vi "fpga_ResamlingCore.vi"(0 "data in":i32, 1 "Channel number":u8, 2 "timestamp":fxp<+,64,32> format="%.42g", 5 "input data valid":bool, 7 "reference in":fxp<+/-,24,3>, 9 "input reference valid":bool, 11 "interpolation factor":u16=192, 12 "Ready for output":bool, 13 "Fnom":T1 items=["Fnom=50Hz", "Fnom=60Hz"]) -> (4 "Resample data and time":T2, 8 "resampling valid":bool, 10 "output valid":bool, 14 "Ready for reference input":bool, 15 "FIFO timeout?":bool)   [LabVIEW 2011, in "NI_EP_Resample_FPGA.lvlib"]
uses:
  <vilib>/addons/Electrical Power/PQ/Resampling/NI_EP_Resample_FPGA.lvlib
  <vilib>/addons/Electrical Power/PQ/Resampling/FPGA/subVIs/fpga_Resampled.ctl
  <vilib>/addons/Electrical Power/PQ/Resampling/FPGA/subVIs/fpga_Typedef Fnom.ctl
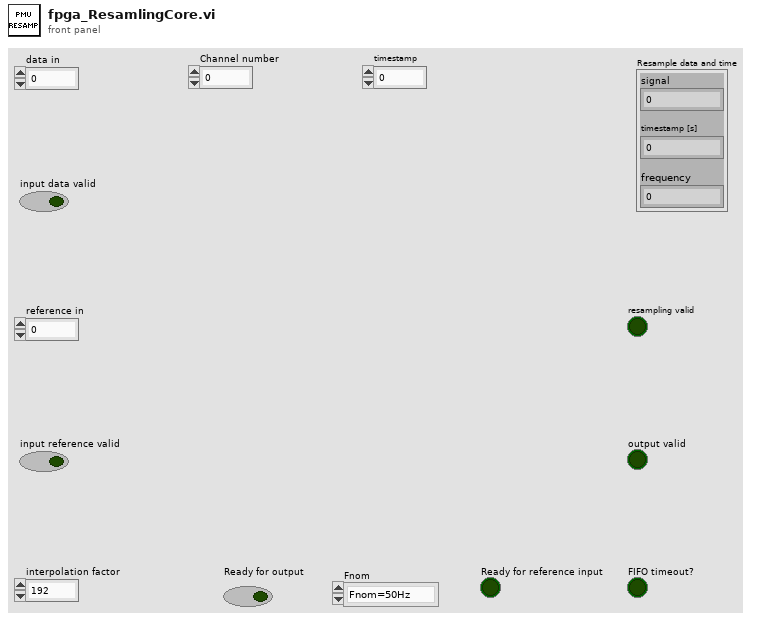
[diagram p1: front panel]
types:
  T1 = typedef "NI_EP_Resample_FPGA.lvlib/fpga_Typedef Fnom.ctl" = u8
  T2 = typedef "NI_EP_Resample_FPGA.lvlib/fpga_Resampled.ctl" = cluster{"signal":fxp<+/-,32,3>, "timestamp [s]":fxp<+,64,32>, "frequency":fxp<+,32,8>}
  T3 = cluster{"bufsize":u16, "bufsize-1":u16, "NChan":u8, "NChan-1":u8, "1/2SymPeriods":i8, "Neg1/2SymPeriods":i8, "polyOrder-1":u8, "maxDec-1":u8}
  T4 = cluster{"TAI timestamp":fxp<+,64,32>, "AI Count":u16}
  T5 = cluster{"even-angle signal":fxp<+/-,32,3>, "Resample position":fxp<+,64,16>, "frequency":fxp<+,32,8>}
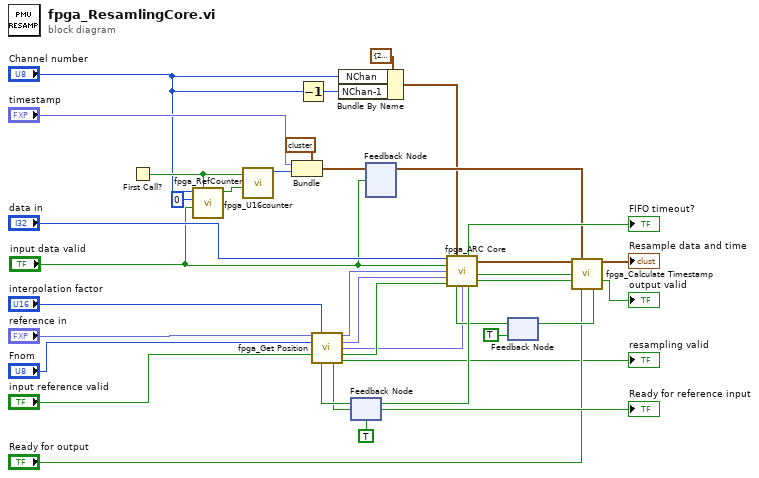
[diagram p0: block diagram]
diagram:
  n1 = First Call?() -> (First Call?: T/F=w11:bool)
  n2 = call <vilib>:"fpga_RefCounter.vi"("reset"=w11, "input valid?"="input data valid", "Reference index"=u8 0, "NChan"="Channel number") -> ("Multichannel enable"=w12:bool)  [unwired: 6 in, 1 out]
  n3 = call <vilib>:"fpga_U16counter.vi"("input valid"=w12, "reset"=w11) -> ("Counter"=w3:u16)  [unwired: 9 in]
  n4 = Bundle(cluster=T4 {"TAI timestamp"=0.0, "AI Count"=0} ("Time count"), "TAI timestamp"="timestamp", "AI Count"=w3) -> (w9:T4)
  n5 = Decrement(x="Channel number") -> (x-1=w14:u8)
  n6 = Bundle By Name(cluster=T3 {"bufsize"=256, "bufsize-1"=255, "NChan"=8, "NChan-1"=7, "1/2SymPeriods"=12, "Neg1/2SymPeriods"=-12, "polyOrder-1"=5, "maxDec-1"=24} ("ARC Constants"), "NChan"="Channel number", "NChan-1"=w14) -> (w6:T3)
  n7 = feedback #1(TRUE ("ready for input")) -> (w33:bool)
  n8 = call <vilib>:"fpga_Get Position.vi"("tach input"="reference in", "Interpolation factor"="interpolation factor", "Fnom"="Fnom", "input valid"="input reference valid", "ready for output"=w33) -> ("resample position [U64.16]"=w26:fxp<+,64,16>, "stepsize [U64.8]"=w27:fxp<+,64,8>, "frequency"=w4:fxp<+,32,8>, "output valid"=w28:bool, "Ready for input"=→"Ready for reference input":bool, "resampling valid"=→"resampling valid":bool)  [unwired: 5 in]
  n9 = feedback #2() -> (w24:T4)  [unwired: 1 in]
  n10 = feedback-in #2(w9, "input data valid") -> ()
  n11 = feedback #3(TRUE ("ready for input")) -> (w20:bool)
  n12 = call <vilib>:"fpga_ARC Core.vi"("data input"="data in", "ARC Constants"=w6, "data valid"="input data valid", "resample position [U64.16]"=w26, "stepsize [U64.8]"=w27, "position valid"=w28, "Ready for output"=w20, "Frequency"=w4) -> ("FIFO timeout?"=→"FIFO timeout?":bool, "resample data"=w25:T5, "muti_ch position valid?"=w23:bool, "ready for input"=w34:bool, "output valid"=w22:bool)  [unwired: 3 in]
  n13 = feedback-in #1(w34) -> ()
  n14 = call <vilib>:"fpga_Calculate Timestamp.vi"("resample data and position"=w25, "timestamp&count"=w24, "muti_ch position valid?"=w23, "input valid"=w22, "ready for output"="Ready for output") -> ("Resample data and time"=→"Resample data and time":T2, "output valid"=→"output valid":bool, "ready for input"=w21:bool)  [unwired: 8 in]
  n15 = feedback-in #3(w21) -> ()
